vi "Status Created Queues.vi"(11 "Queue in":refnum<class "Queue.lvclass">) -> (0 "Created Queue Count":i32, 1 "Created Queue Aliases":string[](array[string]), 2 "Created Queue Exist?":bool, 3 "Queue out":refnum<class "Queue.lvclass">)   [LabVIEW 2021, in "jettl.lvlib" / "Queue.lvclass"]
uses:
  Queue.lvclass
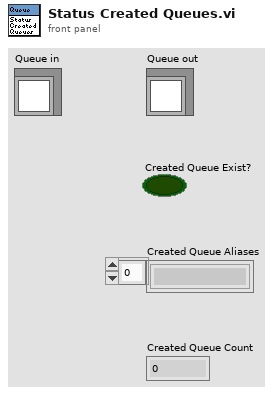
[diagram p1: front panel]
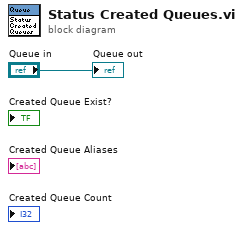
[diagram p0: block diagram]
diagram:
  "Queue out" <- "Queue in"
